vi "main.vi"   [LabVIEW 2020]
types:
  T1 = typedef "game_player.ctl" = cluster{"Name":string, "Winnings":dbl}
  T2 = typedef "queueBus.ctl" = cluster{"UI->Game":refnum<queue>, "UI->Logger":refnum<queue>, "Game -> Logger":refnum<queue>}
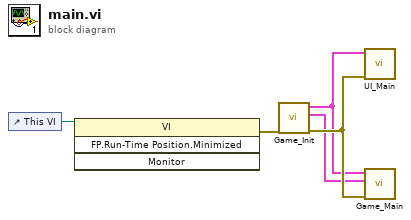
[diagram p0: block diagram]
diagram:
  n1 = control-ref of="This VI"() -> (w2:refnum<vi>)
  n2 = invoke class="VI" method="FP.Run-Time Position.Minimized"(reference=w2) -> (error out=w1:errorcluster)  [unwired: 3 in, 3 out]
  n3 = call "Game_Init.vi"("error in (no error)"=w1) -> ("error out"=w5:errorcluster, "Players array"=w3:T1[], "Queue Bus OUT"=w4:T2)  [unwired: 8 in]
  n4 = call "UI_Main.vi"("error in (no error)"=w5, "Queue Bus"=w4) -> ()  [unwired: 9 in, 1 out]
  n5 = call "Game_Main.vi"("error in (no error)"=w5, "Players array"=w3, "Queue Bus"=w4) -> ()  [unwired: 8 in, 1 out]
